vi "Read Save Image.lvclass.vi"(8 "error in (no error)":errorcluster, 11 "Image Constructor in":refnum<class "Image Constructor.lvclass">) -> (0 "error out":errorcluster, 2 "Save Image.lvclass":refnum<class "Save Image.lvclass">, 3 "Image Constructor out":refnum<class "Image Constructor.lvclass">)   [LabVIEW 2018, in "Image Constructor.lvclass"]
uses:
  Image Constructor.lvclass
  Save Image/Save Image.lvclass
  Image Constructor.lvclass/Image Constructor.ctl
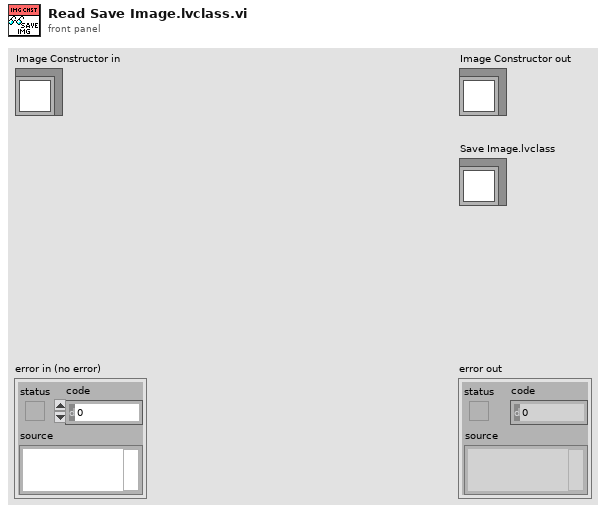
[diagram p1: front panel]
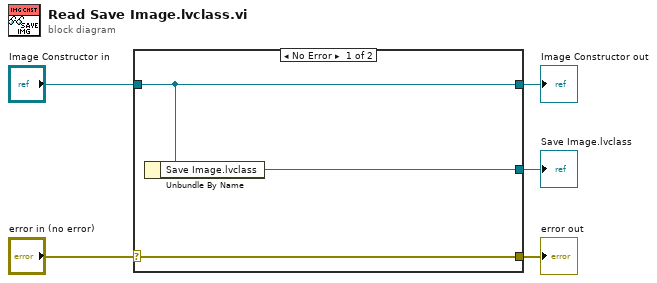
[diagram p0: block diagram]
diagram:
  n1 = case shown="No Error" "error in (no error)" {
    selector: "error in (no error)" -> [w8 w9]
    tunnel: [w8 w9] -> w4
    tunnel: [w7 w10] -> w2
    tunnel: "Image Constructor in" -> [w7 w10]
    tunnel: [w6 _] -> w1
    frame No Error {
      n2 = Unbundle By Name(w7) -> ("Save Image.lvclass"=w6:refnum<class "Save Image.lvclass">)
    }
    frame Error {
    }
  }
  "error out" <- w4
  "Image Constructor out" <- w2
  "Save Image.lvclass" <- w1
